vi "GetStageStopped.vi"(8 "error in":errorcluster, 9 "Stage":T1, 11 "reference in":refnum<k7>) -> (0 "error out":errorcluster, 2 "Stage Position":string, 3 "reference out":refnum<k7>)   [LabVIEW 2020]
uses:
  StageSelector--Enum.ctl
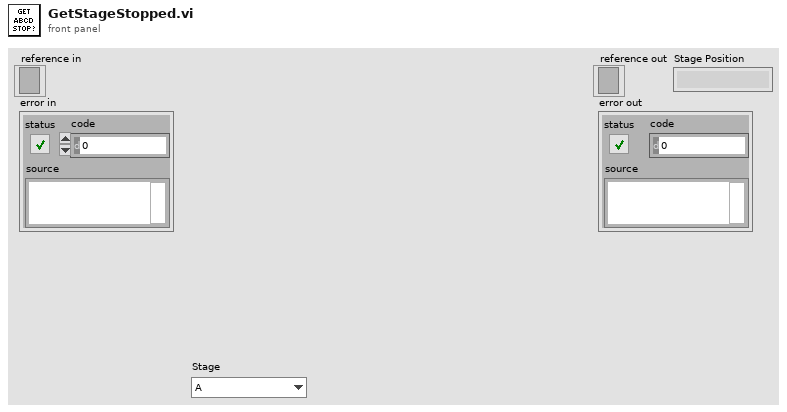
[diagram p1: front panel]
types:
  T1 = typedef "StageSelector--Enum.ctl" = enum16{"A", "B", "C", "D"}
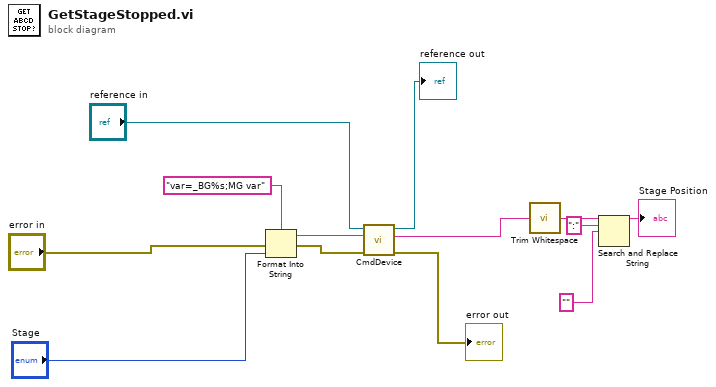
[diagram p0: block diagram]
diagram:
  n1 = Format Into String(format string="var=_BG%s;MG var", error in="error in", "Stage") -> (resulting string=w3:string, error out=w11:errorcluster)  [unwired: 1 in]
  n2 = call "CmdDevice.vi"("error in (no error)"=w11, "Command:"=w3, "reference in"="reference in") -> ("error out"=→"error out":errorcluster, "Response:"=w5:string, "reference out"=→"reference out":refnum<k7>)  [unwired: 6 in]
  n3 = call <vilib>:"Trim Whitespace.vi"("string"=w5) -> ("trimmed string"=w8:string)  [unwired: 1 in]
  n4 = Search and Replace String(input string=w8, search string=":", replace string="" ("replace string (\"\")")) -> (result string=→"Stage Position":string)  [unwired: 5 in, 3 out]
